vi "End ClientStreamTemplate.vi"(8 "error in":errorcluster, 11 "Call ID in":T2) -> (0 "error out":errorcluster, 1 "errorDetails":T1, 2 "Response Data":cluster{"Numeric":dbl})   [LabVIEW 2019, in "Client Template.lvlib"]
uses:
  Client Template.lvlib
  gRPC lv Support/Shared/grpcId.ctl
  gRPC lv Support/Shared/Any.ctl
  2435b599-b0f7-48e4-804e-62ee509d3e35.vi
  9ddb346c-f848-4ec1-9569-72f30e6bd646.vi
  gRPC lv Support/Shared/TranslateGrpcError.vi
  gRPC lv Support/Shared/Wait On Occurrence.vi
  gRPC lv Support/Shared/Is Feature Enabled.vi
  gRPC lv Support/Server API/Server/Get Server DLL Path.vi
  <vilib>/Utility/error.llb/Error Cluster From Error Code.vi
  gRPC lv Support/grpc-lvsupport.lvlib
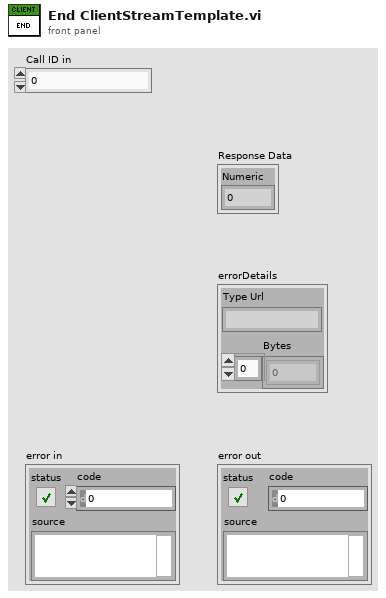
[diagram p1: front panel]
types:
  T1 = typedef "grpc-lvsupport.lvlib/Any.ctl" = cluster{"Type Url":string, "Bytes":u8[]}
  T2 = typedef "grpc-lvsupport.lvlib/grpcId.ctl" = u64
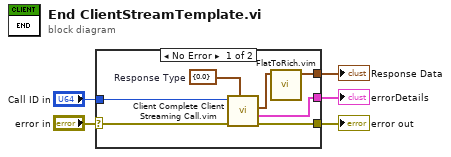
[diagram p0: block diagram]
diagram:
  n1 = case shown="No Error" "error in" {
    selector: "error in" -> [w12 w13]
    tunnel: [w11 w13] -> w4
    tunnel: "Call ID in" -> [w10 _]
    tunnel: [w6 _] -> w2
    tunnel: [w8 _] -> w1
    frame No Error {
      w9 = cluster{"Numeric":dbl} {"Numeric"=0.0}  # Response Type
      n2 = call "Client Complete Client Streaming Call.vim"("Response Type"=w9, "error in"=w12, "Call ID in"=w10) -> ("error out"=w11:errorcluster, "errorDetails"=w8:T1, "Response Data"=w7:cluster{"Numeric":dbl})  [unwired: 6 in]
      n3 = call "FlatToRich.vim"("InputCluster"=w7) -> ("OutputCluster"=w6:cluster{"Numeric":dbl})  [unwired: 10 in]
    }
    frame Error {
    }
  }
  "error out" <- w4
  "Response Data" <- w2
  "errorDetails" <- w1
